vi "EnableCell.vi"(0 "MenuDisableCol in":refnum<class "MenuDisableCol.lvclass">, 1 "Col Array Ref in":refnum<vi>, 5 "Cell Position":T1, 7 "Table Data in":string[][](array[string]), 9 "Table CtlRef In":refnum<vi>, 11 "error in (no error)":errorcluster) -> (4 "MenuDisableCol out":refnum<class "MenuDisableCol.lvclass">, 8 "Table Data out":string[][](array[string]), 10 "Table CtlRef Out":refnum<vi>, 15 "error out":errorcluster)   [LabVIEW 2013, in "MenuDisableCol.lvclass"]
uses:
  MenuDisableCol.lvclass
  <vilib>/Utility/miscctls.llb/LVRowAndColumnTypeDef.ctl
  MenuCol/MenuCol.lvclass
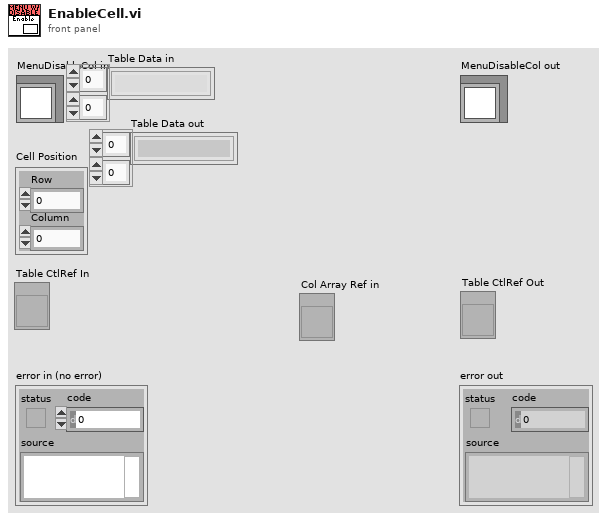
[diagram p1: front panel]
types:
  T1 = typedef "LVRowAndColumnTypeDef.ctl" = cluster{"Row":i32, "Column":i32}
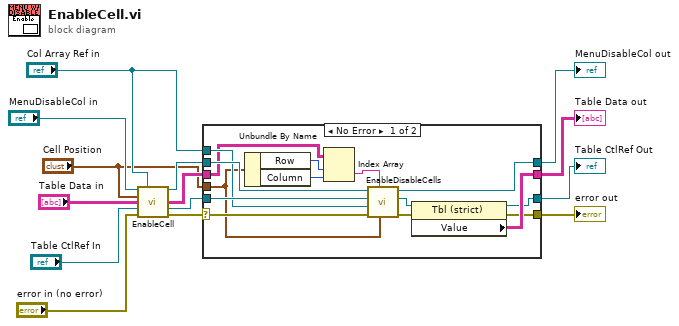
[diagram p0: block diagram]
diagram:
  n1 = call-parent "EnableCell.vi"("Column in"="MenuDisableCol in", "Col Array Ref in"="Col Array Ref in", "Cell Position"="Cell Position", "Table Data in"="Table Data in", "Table CtlRef In"="Table CtlRef In", "error in (no error)"="error in (no error)") -> ("Column out"=w2:refnum<class "MenuDisableCol.lvclass">, "Table Data out"=w3:string[][], "Table CtlRef Out"=w4:refnum<vi>, "error out"=w5:errorcluster)  [unwired: 6 in]
  n2 = case shown="No Error" w5 {
    selector: w5 -> [w20 w32]
    tunnel: "Cell Position" -> [w18 _]
    tunnel: "Col Array Ref in" -> [w21 _]
    tunnel: w2 -> [w26 w31]
    tunnel: [w29 w33] -> w9
    tunnel: [w28 w32] -> w7
    tunnel: [w27 w30] -> w8
    tunnel: [w23 w31] -> w6
    tunnel: w3 -> [w19 w33]
    tunnel: w4 -> [w22 w30]
    frame No Error {
      n3 = Unbundle By Name(w18) -> ("Row"=w17:i32, "Column"=w16:i32)
      n4 = Index Array(array=w19, index (row)=w17, index (col)=w16) -> (element=w15:string)
      n5 = call-dynamic "EnableDisableCells.vi"("Cell Position"=w18, "Item Name or Tag"=w15, "error in (no error)"=w20, "Col Array Ref in"=w21, "Table CtlRef in"=w22, "MenuDisableCol in"=w26) -> ("error out"=w25:errorcluster, "Table CtlRef out"=w24:refnum<vi>, "MenuDisableCol out"=w23:refnum<class "MenuDisableCol.lvclass">)  [unwired: 2 in, 1 out]
      n6 = property class="Tbl (strict)"(reference=w24, error in=w25) -> (reference out=w27:refnum<vi>, error out=w28:errorcluster, "Value"=w29:string[][])
    }
    frame Error {
    }
  }
  "error out" <- w7
  "MenuDisableCol out" <- w6
  "Table CtlRef Out" <- w8
  "Table Data out" <- w9
